vi "LinearSystemLoop_Execute.vi"(5 "Linear System":T2, 7 "LinearSystemLoop_Control_Params":T1, 8 "dT_Seconds":dbl=0.02 format="%#_13g", 10 "ProcessVariables":dbl[](array[numeric]), 11 "Setpoints":dbl[](array[numeric])) -> (0 "Error":bool, 2 "Filtered Measurements":dbl[](array[numeric]), 3 "ControlOutputs":dbl[](array[numeric]), 4 "out Linear System Loop":T4)   [LabVIEW 2019, in "Trajectory_Library.lvlib"]
uses:
  Trajectory_Library.lvlib
  TypeDef/LINEAR_SYSTEM_LOOP.ctl
  TypeDef/LINEAR_QUADRATIC_REGULATOR.ctl
  <vilib>/Analysis/Matrix/Datatypes/RealMatrix.ctl
  TypeDef/LINEAR_PLANT_INV_FF.ctl
  TypeDef/KALMAN_FILTER.ctl
  TypeDef/LINEAR_SYSTEM.ctl
  TypeDef/LINEAR_SYSTEM_LOOP_CTRL_PARAMS.CTL
  MatBuilder_Create.vi
  <vilib>/Analysis/Matrix/Numeric/Conversions/Array To Matrix - RA.vi
  <vilib>/Analysis/Matrix/Numeric/Conversions/Matrix To Array - RM.vi
  <vilib>/Analysis/Matrix/NI_Matrix.lvlib
panel:
  # "<States,States>"
  # "<States,Inputs>"
  # "<Outputs,States>"
  # "<Outputs,Inputs>"
  # "<States,1>"
  # "<FUTURE --- CLAMP TYPE -- For now\nuse Normalize>"
  # "Steady State Gain  \n<States,Outputs>"
  # "State Estimate <Statess,1>"
  # "<States,States>"
  # "<States,Inputs>"
  # "<Outputs,States>"
  # "<Outputs,Inputs>"
  # "<States,1>"
  # "<Inputs,1>"
  # "<States,Inputs>"
  # "<States,States>"
  # "Ref State <States,1>"
  # "Comp and capped \noutput <Inputs,1>"
  # "Controller gain\n<Inputs,States>"
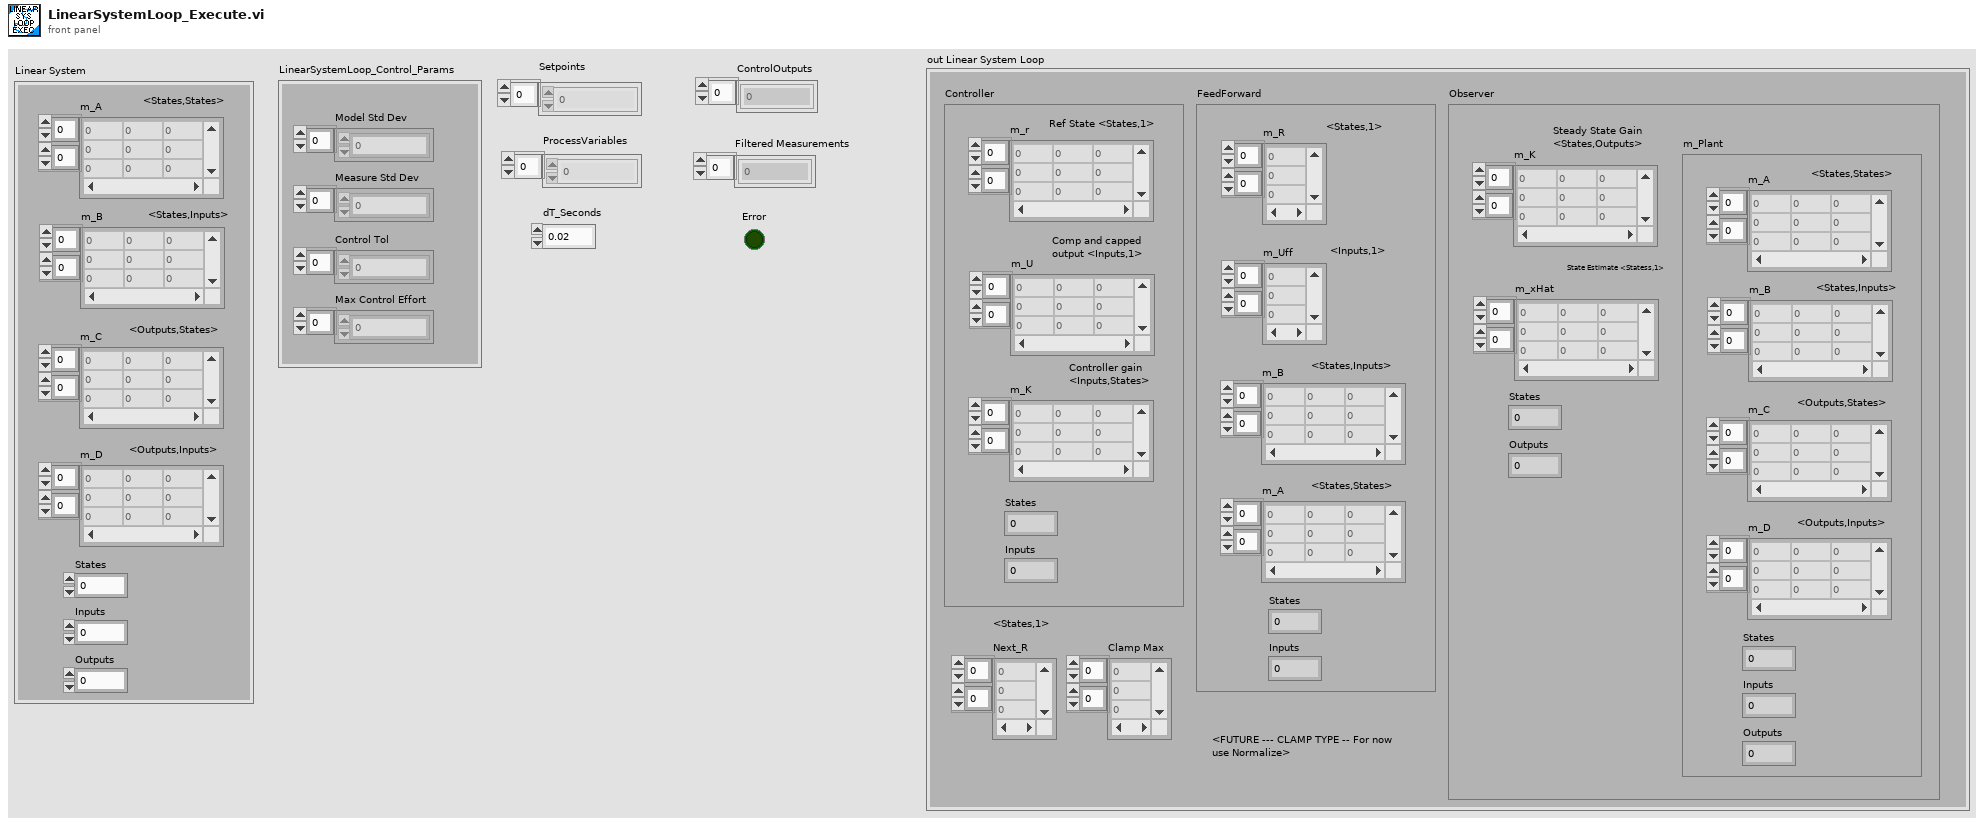
[diagram p1: front panel]
types:
  T1 = typedef "Trajectory_Library.lvlib/LINEAR_SYSTEM_LOOP_CTRL_PARAMS.CTL" = cluster{"Model Std Dev":dbl[], "Measure Std Dev":dbl[], "Control Tol":dbl[], "Max Control Effort":dbl[]}
  T2 = typedef "Trajectory_Library.lvlib/LINEAR_SYSTEM.ctl" = cluster{"m_A":T3, "m_B":T3, "m_C":T3, "m_D":T3, "States":i32, "Inputs":i32, "Outputs":i32}
  T3 = typedef "NI_Matrix.lvlib/RealMatrix.ctl" = dbl[][]
  T4 = typedef "Trajectory_Library.lvlib/LINEAR_SYSTEM_LOOP.ctl" = cluster{"Controller":T5, "FeedForward":T6, "Observer":T7, "Next_R":T3, "Clamp Max":T3}
  T5 = typedef "Trajectory_Library.lvlib/LINEAR_QUADRATIC_REGULATOR.ctl" = cluster{"m_r":T3, "m_U":T3, "m_K":T3, "States":i32, "Inputs":i32}
  T6 = typedef "Trajectory_Library.lvlib/LINEAR_PLANT_INV_FF.ctl" = cluster{"m_R":T3, "m_Uff":T3, "m_B":T3, "m_A":T3, "States":i32, "Inputs":i32}
  T7 = typedef "Trajectory_Library.lvlib/KALMAN_FILTER.ctl" = cluster{"m_K":T3, "m_xHat":T3, "States":i32, "Outputs":i32, "m_Plant":T2}
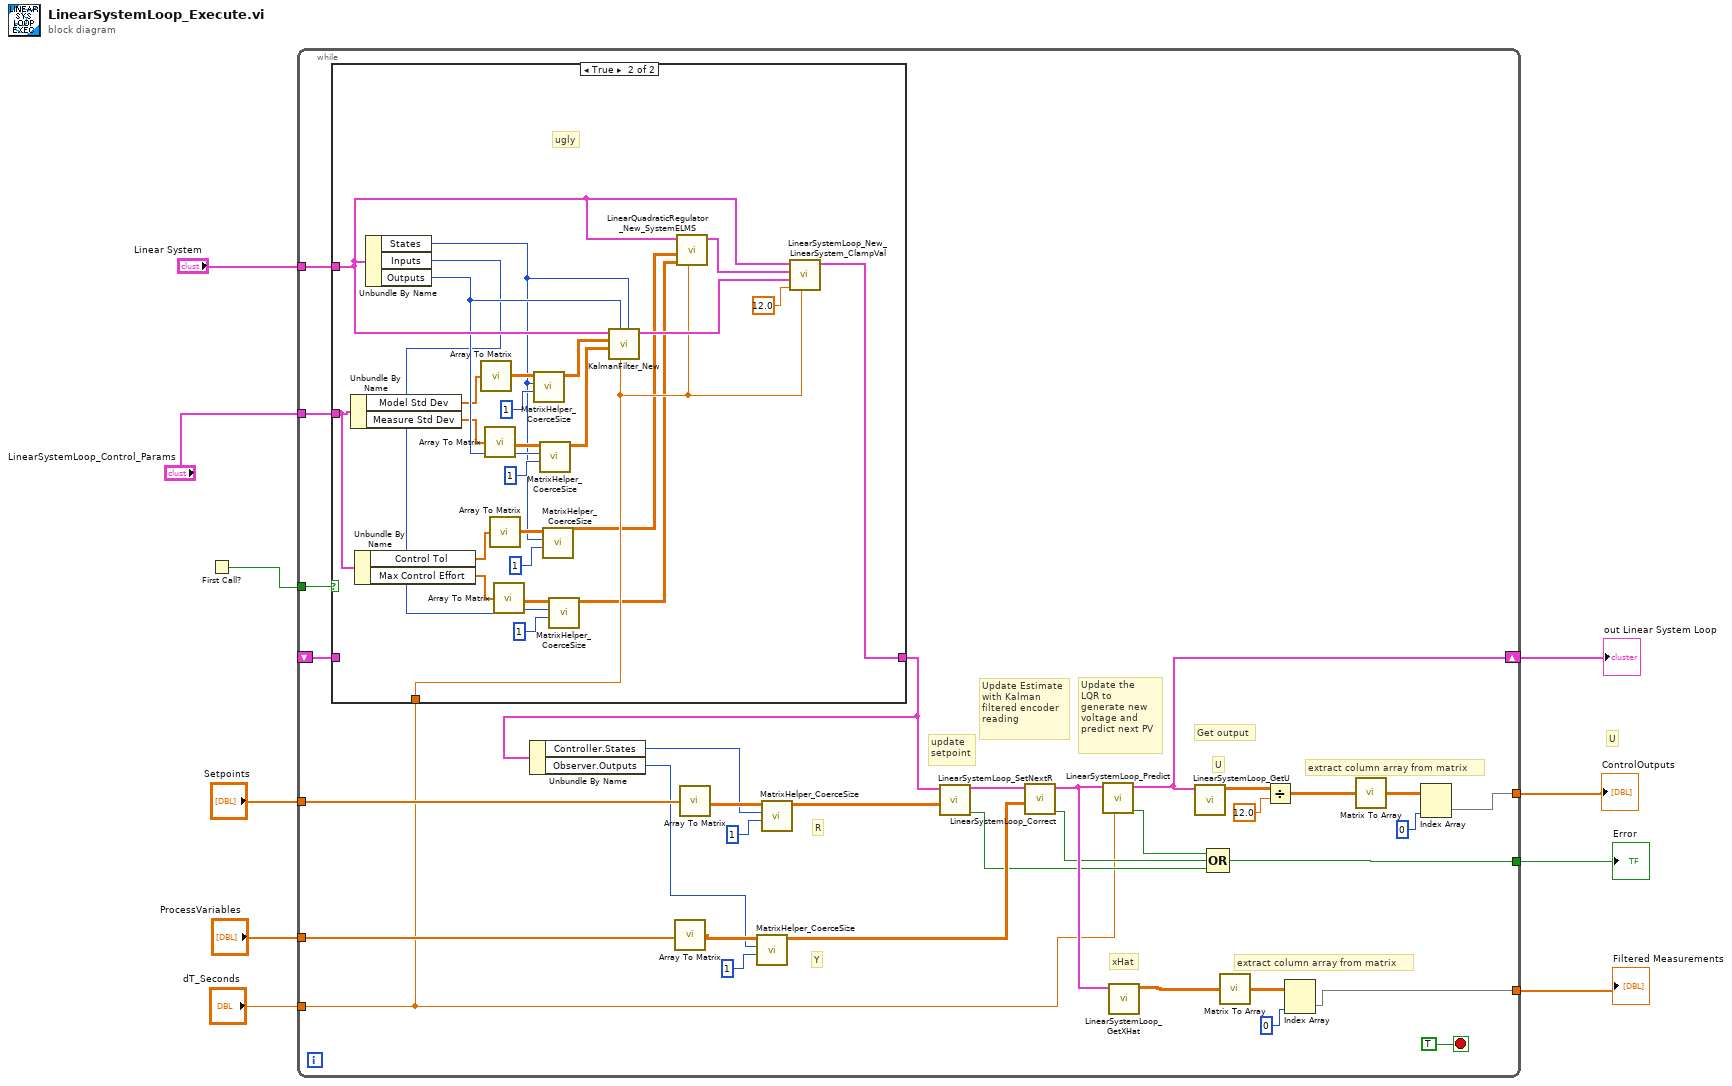
[diagram p0: block diagram]
diagram:
  # "U"
  n1 = First Call?() -> (First Call?: T/F=w6:bool)
  n2 = while {
    tunnel: [w39] -> w9
    tunnel: [w19] -> w4
    tunnel: "Setpoints" -> [w35]
    tunnel: "ProcessVariables" -> [w30]
    shift-right: [w43] -> w10
    shift-left: _ -> [w13]
    tunnel: w6 -> [w28]
    tunnel: [w23] -> w5
    tunnel: "dT_Seconds" -> [w14]
    tunnel: "Linear System" -> [w15]
    tunnel: "LinearSystemLoop_Control_Params" -> [w11]
    stop <- TRUE stop-if-true
    # "extract column array from matrix"
    # "extract column array from matrix"
    # "xHat"
    # "U"
    # "Y"
    # "R"
    # "Get output"
    # "Update the \nLQR to \ngenerate new \nvoltage and \npredict next PV"
    # "update \nsetpoint"
    # "Update Estimate\nwith Kalman \nfiltered encoder \nreading"
    n3 = case shown="True" w28 {
      tunnel: [w45 w67] -> w12
      tunnel: w13 -> [w45 _]
      tunnel: w15 -> [_ w70]
      tunnel: w14 -> [_ w66]
      tunnel: w11 -> [_ w50]
      frame False {
      }
      frame True {
        # "ugly"
        n4 = Unbundle By Name(w50) -> ("Model Std Dev"=w60:dbl[], "Measure Std Dev"=w59:dbl[])
        n5 = Unbundle By Name(w50) -> ("Control Tol"=w52:dbl[], "Max Control Effort"=w51:dbl[])
        n6 = Unbundle By Name(w70) -> ("States"=w49:i32, "Inputs"=w48:i32, "Outputs"=w61:i32)
        n7 = call-poly <vilib>:"Array To Matrix.vi"("Real 1D Array"=w60) -> ("Real Matrix (Column Vector)"=w64:T3)
        n8 = call-poly <vilib>:"Array To Matrix.vi"("Real 1D Array"=w59) -> ("Real Matrix (Column Vector)"=w62:T3)
        n9 = call-poly <vilib>:"Array To Matrix.vi"("Real 1D Array"=w52) -> ("Real Matrix (Column Vector)"=w55:T3)
        n10 = call-poly <vilib>:"Array To Matrix.vi"("Real 1D Array"=w51) -> ("Real Matrix (Column Vector)"=w53:T3)
        n11 = call "MatrixHelper_CoerceSize.vi"("Columns"=1, "Rows"=w49, "input matrix"=w64) -> ("output matrix"=w58:T3)  [unwired: 7 in, 1 out]
        n12 = call "MatrixHelper_CoerceSize.vi"("Columns"=1, "Rows"=w61, "input matrix"=w62) -> ("output matrix"=w57:T3)  [unwired: 7 in, 1 out]
        n13 = call "MatrixHelper_CoerceSize.vi"("Columns"=1, "Rows"=w49, "input matrix"=w55) -> ("output matrix"=w47:T3)  [unwired: 7 in, 1 out]
        n14 = call "MatrixHelper_CoerceSize.vi"("Columns"=1, "Rows"=w48, "input matrix"=w53) -> ("output matrix"=w46:T3)  [unwired: 7 in, 1 out]
        n15 = call "KalmanFilter_New.vi"("States"=w49, "dt_Seconds"=w66, "Outputs"=w61, "MeasurementStdDevs"=w57, "StateStdDevs"=w58, "Plant"=w70) -> ("KalmanFilter"=w69:T7)  [unwired: 4 in, 1 out]
        n16 = call "LinearQuadraticRegulator_New_SystemELMS.vi"("dt_Seconds"=w66, "Relms"=w46, "Qelms"=w47, "LINEARSYSTEM"=w70) -> ("LinearQuadraticRegulator"=w71:T5)  [unwired: 6 in, 1 out]
        n17 = call "LinearSystemLoop_New_LinearSystem_ClampVal.vi"("dT_Seconds"=w66, "Max_Voltage"=12.0, "Observer"=w69, "Controller"=w71, "Plant"=w70) -> ("Linear System Loop"=w67:T4)  [unwired: 5 in, 1 out]
      }
    }
    n18 = Unbundle By Name(w12) -> ("Controller.States"=w27:i32, "Observer.Outputs"=w26:i32)
    n19 = call-poly <vilib>:"Array To Matrix.vi"("Real 1D Array"=w30) -> ("Real Matrix (Column Vector)"=w31:T3)
    n20 = call-poly <vilib>:"Array To Matrix.vi"("Real 1D Array"=w35) -> ("Real Matrix (Column Vector)"=w34:T3)
    n21 = call "MatrixHelper_CoerceSize.vi"("Columns"=1, "Rows"=w26, "input matrix"=w31) -> ("output matrix"=w29:T3)  [unwired: 7 in, 1 out]
    n22 = call "MatrixHelper_CoerceSize.vi"("Columns"=1, "Rows"=w27, "input matrix"=w34) -> ("output matrix"=w33:T3)  [unwired: 7 in, 1 out]
    n23 = call "LinearSystemLoop_SetNextR.vi"("R"=w33, "input inear System Loop"=w12) -> ("Size Coerced"=w16:bool, "out Linear System Loop"=w44:T4)  [unwired: 8 in]
    n24 = call "LinearSystemLoop_Correct.vi"("Y"=w29, "input inear System Loop"=w44) -> ("Error"=w40:bool, "out Linear System Loop"=w42:T4)  [unwired: 8 in]
    n25 = call "LinearSystemLoop_Predict.vi"("dT_Seconds"=w14, "input inear System Loop"=w42) -> ("Error"=w41:bool, "out Linear System Loop"=w43:T4)  [unwired: 8 in]
    n26 = call "LinearSystemLoop_GetXHat.vi"("input inear System Loop"=w42) -> ("XHat"=w17:T3)  [unwired: 10 in]
    n27 = call "LinearSystemLoop_GetU.vi"("input inear System Loop"=w43) -> ("U"=w38:T3)  [unwired: 10 in]
    n28 = Compound Arithmetic op=OR(w41, w40, w16) -> (w39:bool)
    n29 = call-poly <vilib>:"Matrix To Array.vi"("Real Matrix"=w17) -> ("Real 2D Array"=w25:dbl[][])
    n30 = Divide(x=w38, y=12.0) -> (x/y=w20:T3)
    n31 = Index Array(array=w25, index (col)=0 ("disabled index (col)")) -> (element=w23:dbl[])  [unwired: 1 in]
    n32 = call-poly <vilib>:"Matrix To Array.vi"("Real Matrix"=w20) -> ("Real 2D Array"=w22:dbl[][])
    n33 = Index Array(array=w22, index (col)=0 ("disabled index (col)")) -> (element=w19:dbl[])  [unwired: 1 in]
  }
  "out Linear System Loop" <- w10
  "Error" <- w9
  "Filtered Measurements" <- w5
  "ControlOutputs" <- w4
